vi "VirtualBench_Set_TestVerdict.vi"(11 "WaveformResultAnalysis":bool) -> (0 "error out":errorcluster, 2 "Report Text":string, 3 "Test Result":bool)   [LabVIEW 2016]
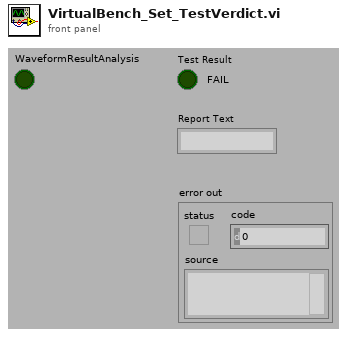
[diagram p1: front panel]
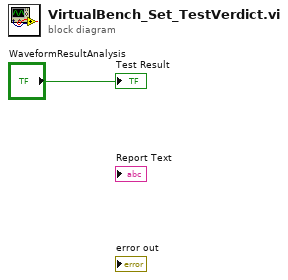
[diagram p0: block diagram]
diagram:
  "Test Result" <- "WaveformResultAnalysis"
